vi "Const Configuration Default.vi"() -> (3 "Config":T1={"Language"={"Name"="English"}, "Path Config"={"Data Folder Path"=path "", "PNG Folder Path"=path "", "mp3 Folder Path"=path ""}, "Image Viewer Config"={"Center Point"={"Size"=3, "Color"=16448250, "Show?"=TRUE}, "bp Point"={"Size"=3, "Color"=16711680, "Show?"=TRUE}, "w Point"={"Size"=3, "Color"=10546431, "Show?"=TRUE}, "b Box"={"Fill Color"=16752543, "Border Color"=16752543, "Show?"=TRUE}, "i Box"={"Fill Color"=16776305, "Border Color"=16776305, "Show?"=TRUE}, "o Point"={"Size"=3, "Color"=10546431, "Show?"=TRUE}, "c Point"={"Size"=3, "Color"=10546431, "Show?"=TRUE}}})   [LabVIEW 2018, in "Main Panel.lvlib" / "Main Panel.lvclass"]
uses:
  Main Panel.lvclass
  Const Configuration.ctl
  Const Path Setting.ctl
  Const Image Viewer Setting.ctl
  Framework/Framework/Framework.lvclass
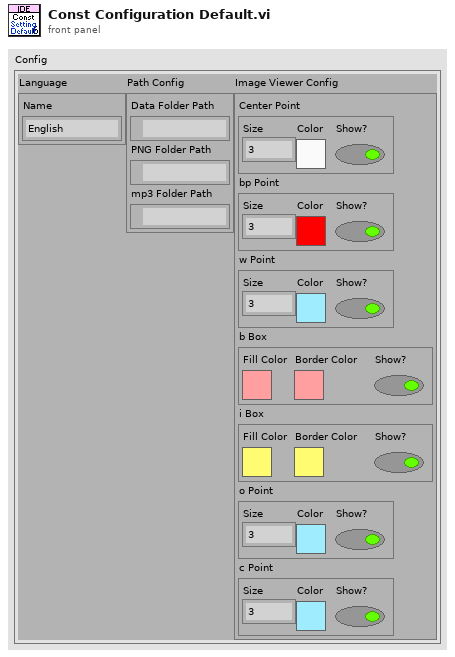
[diagram p1: front panel]
types:
  T1 = typedef "Main Panel.lvlib/Main Panel.lvclass/Const Configuration.ctl" = cluster{"Language":cluster{"Name":string}, "Path Config":T2, "Image Viewer Config":T3}
  T2 = typedef "Main Panel.lvlib/Main Panel.lvclass/Const Path Setting.ctl" = cluster{"Data Folder Path":path, "PNG Folder Path":path, "mp3 Folder Path":path}
  T3 = typedef "Main Panel.lvlib/Main Panel.lvclass/Const Image Viewer Setting.ctl" = cluster{"Center Point":cluster{"Size":i32, "Color":u32, "Show?":bool}, "bp Point":cluster{"Size":i32, "Color":u32, "Show?":bool}, "w Point":cluster{"Size":i32, "Color":u32, "Show?":bool}, "b Box":cluster{"Fill Color":u32, "Border Color":u32, "Show?":bool}, "i Box":cluster{"Fill Color":u32, "Border Color":u32, "Show?":bool}, "o Point":cluster{"Size":i32, "Color":u32, "Show?":bool}, "c Point":cluster{"Size":i32, "Color":u32, "Show?":bool}}
  T4 = cluster{"LF2R Path":path, "Data Path":path, "PNG Path":path, "mp3 Path":path}
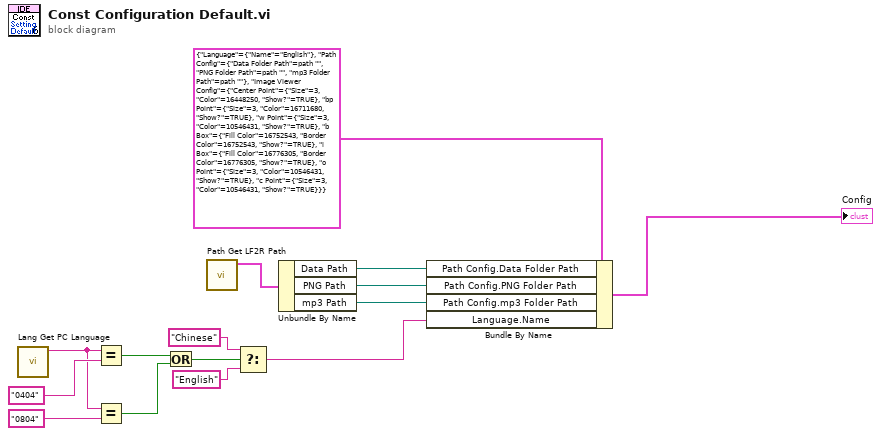
[diagram p0: block diagram]
diagram:
  n1 = call "Lang Get PC Language.vi"() -> ("Language Hex Code"=w12:string)  [unwired: 11 in]
  n2 = Equal?(x=w12, y="0404") -> (x = y?=w10:bool)
  n3 = Equal?(x=w12, y="0804") -> (x = y?=w9:bool)
  n4 = Or(x=w10, y=w9) -> (x .or. y?=w8:bool)
  n5 = call "Path Get LF2R Path.vi"() -> ("Path"=w4:T4)  [unwired: 9 in, 2 out]
  n6 = Select(t="Chinese" ("y"), s=w8, f="English" ("y")) -> (s? t:f=w5:string)
  n7 = Unbundle By Name(w4) -> ("Data Path"=w3:path, "PNG Path"=w2:path, "mp3 Path"=w1:path)
  n8 = Bundle By Name(cluster=T1 {"Language"={"Name"="English"}, "Path Config"={"Data Folder Path"=path "", "PNG Folder Path"=path "", "mp3 Folder Path"=path ""}, "Image Viewer Config"={"Center Point"={"Size"=3, "Color"=16448250, "Show?"=TRUE}, "bp Point"={"Size"=3, "Color"=16711680, "Show?"=TRUE}, "w Point"={"Size"=3, "Color"=10546431, "Show?"=TRUE}, "b Box"={"Fill Color"=16752543, "Border Color"=16752543, "Show?"=TRUE}, "i Box"={"Fill Color"=16776305, "Border Color"=16776305, "Show?"=TRUE}, "o Point"={"Size"=3, "Color"=10546431, "Show?"=TRUE}, "c Point"={"Size"=3, "Color"=10546431, "Show?"=TRUE}}} ("Config 2"), "Path Config.Data Folder Path"=w3, "Path Config.PNG Folder Path"=w2, "Path Config.mp3 Folder Path"=w1, "Language.Name"=w5) -> (→"Config":T1)
